vi "Sort Tree By Column.vi"(8 "error in (no error)":errorcluster, 10 "Col":i32, 11 "Configuration in":T1) -> (0 "error out":errorcluster, 3 "Configuration Out":T1)   [LabVIEW 2013, in "LVTM.lvlib"]
uses:
  LVTM.lvlib
  Controls_LVTM/LVTM_Config_Info.ctl
  Controls_LVTM/View.ctl
  Controls_LVTM/SharedDataDVR.ctl
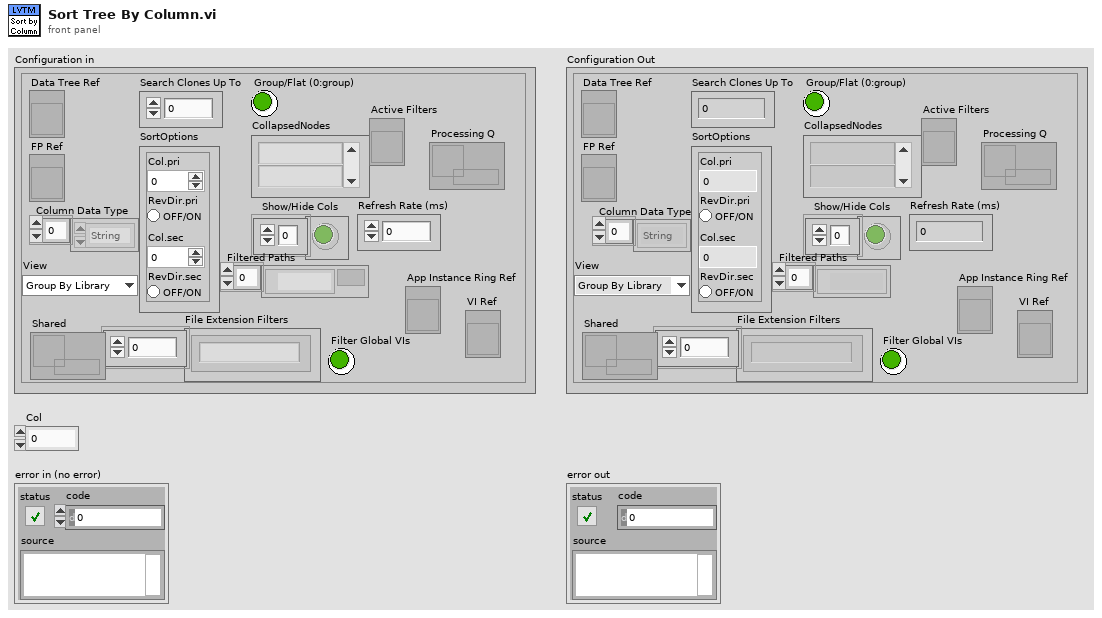
[diagram p1: front panel]
types:
  T1 = typedef "LVTM.lvlib/LVTM_Config_Info.ctl" = cluster{"Data Tree Ref":refnum<vi>, "FP Ref":refnum<vi>, "Column Data Type":enum16{"String", "Numeric"}[], "Search Clones Up To":i32, "SortOptions":cluster{"Col.pri":i32, "RevDir.pri":bool, "Col.sec":i32, "RevDir.sec":bool}, "Group/Flat (0:group)":bool, "CollapsedNodes":string[], "Show/Hide Cols":bool[], "Filtered Paths":path[], "View":T2, "File Extension Filters":string[], "Filter Global VIs":bool, "Shared":refnum<data-value>, "Active Filters":refnum<vi>, "Refresh Rate (ms)":i32, "App Instance Ring Ref":refnum<vi>, "Processing Q":refnum<queue>, "VI Ref":refnum<vi>}
  T2 = typedef "LVTM.lvlib/View.ctl" = enum16{"Group By Library", "Group By Folder", "Flat List"}
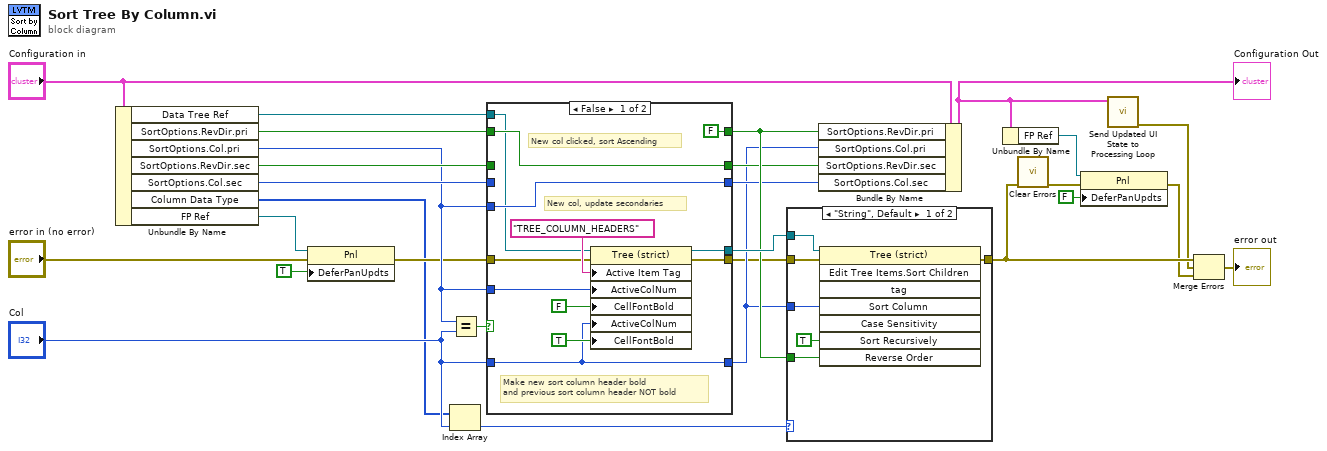
[diagram p0: block diagram]
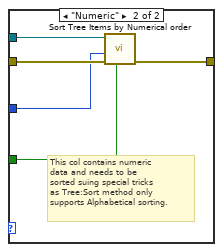
[diagram p2: hidden frame]
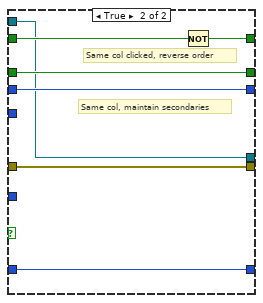
[diagram p3: hidden frame]
diagram:
  n1 = Unbundle By Name("Configuration in") -> ("Data Tree Ref"=w27:refnum<vi>, "SortOptions.RevDir.pri"=w22:bool, "SortOptions.Col.pri"=w23:i32, "SortOptions.RevDir.sec"=w24:bool, "SortOptions.Col.sec"=w25:i32, "Column Data Type"=w12:enum16{"String", "Numeric"}[], "FP Ref"=w18:refnum<vi>)
  n2 = property class="Pnl"(reference=w18, error in="error in (no error)", "DeferPanUpdts"=TRUE ("Defer Panel Updates")) -> (error out=w17:errorcluster)  [unwired: 1 out]
  n3 = Index Array(array=w12, index="Col") -> (element=w14:enum16{"String", "Numeric"})
  n4 = Equal?(x=w23, y="Col") -> (x = y?=w9:bool)
  n5 = case shown="False" w9 {
    tunnel: w22 -> [w32 w43]
    tunnel: [FALSE ("Sorted AZ?") w42] -> w26
    tunnel: w17 -> [w36 w47]
    tunnel: [w35 w47] -> w10
    tunnel: "Col" -> [w34 w46]
    tunnel: [w34 w46] -> w11
    tunnel: w23 -> [w33 _]
    tunnel: [w32 w45] -> w20
    tunnel: w23 -> [w31 _]
    tunnel: [w31 w44] -> w21
    tunnel: w24 -> [_ w45]
    tunnel: w25 -> [_ w44]
    tunnel: w27 -> [w30 w41]
    tunnel: [w29 w41] -> w28
    frame False {
      # "New col, update secondaries"
      # "Make new sort column header bold\nand previous sort column header NOT bold"
      # "New col clicked, sort Ascending"
      n6 = property on="Property Node" class="Tree (strict)"(reference=w30, error in=w36, "Active Item Tag"="TREE_COLUMN_HEADERS" ("Active Item:Tag"), "ActiveColNum"=w33, "CellFontBold"=FALSE ("Active Cell:Cell Font:Bold"), "ActiveColNum"=w34, "CellFontBold"=TRUE ("Active Cell:Cell Font:Bold")) -> (reference out=w29:refnum<vi>, error out=w35:errorcluster)
    }
    frame True {
      # "Same col, maintain secondaries"
      # "Same col clicked, reverse order"
      n7 = Not(x=w43) -> (.not. x?=w42:bool)
    }
  }
  n8 = case shown="\"String\", Default" w14 {
    tunnel: [w53 w57] -> w4
    tunnel: w26 -> [w52 w56]
    tunnel: w10 -> [w51 w58]
    tunnel: w11 -> [w50 w54]
    tunnel: w28 -> [w48 w55]
    frame "String", Default {
      n9 = invoke on="Invoke Node" class="Tree (strict)" method="Edit Tree Items.Sort Children"(reference=w48, error in=w51, "Sort Column"=w50, "Sort Recursively"=TRUE ("Sort Recursively?"), "Reverse Order"=w52) -> (error out=w53:errorcluster)  [unwired: 3 in, 7 out]
    }
    frame "Numeric" {
      # "This col contains numeric\ndata and needs to be\nsorted suing special tricks\nas Tree:Sort method only\nsupports Alphabetical sorting."
      n10 = call "Sort Tree Items by Numerical order.vi"("Reverse Order?"=w56, "error in"=w58, "Sort Column"=w54, "Data Tree"=w55) -> ("error out"=w57:errorcluster)  [unwired: 7 in]
    }
  }
  n11 = Bundle By Name(cluster="Configuration in", "SortOptions.RevDir.pri"=w26, "SortOptions.Col.pri"=w11, "SortOptions.RevDir.sec"=w20, "SortOptions.Col.sec"=w21) -> (w6:T1)
  "Configuration Out" <- w6
  n12 = Unbundle By Name(w6) -> ("FP Ref"=w7:refnum<vi>)
  n13 = call <vilib>:"Clear Errors.vi"("error in (no error)"=w4) -> ("error out"=w5:errorcluster)  [unwired: 6 in]
  n14 = property class="Pnl"(reference=w7, error in=w5, "DeferPanUpdts"=FALSE ("Defer Panel Updates")) -> (error out=w1:errorcluster)  [unwired: 1 out]
  n15 = call "Send Updated UI State to Processing Loop.vi"("ConfigInfo in"=w6) -> ("error out"=w2:errorcluster)  [unwired: 10 in]
  n16 = Merge Errors(w4, w2, w1) -> (→"error out":errorcluster)
